vi "FileSync.Read Config.vi"(8 "error in (no error)":errorcluster, 9 "Dialog":bool, 10 "Config File":path, 11 "File.Sync in":refnum<class "File.Sync.lvclass">) -> (0 "error out":errorcluster, 1 "SyncItems":T1[](array[typedef]), 2 "Saved":bool, 3 "File.Sync out":refnum<class "File.Sync.lvclass">)   [LabVIEW 2024, in "KATE_Lib.lvlib" / "File Utils.lvlib" / "File.Sync.lvclass"]
uses:
  File.Sync.lvclass
  File.Sync Item Record.ctl
  File.Sync.lvclass/File.Sync.ctl
  File Utils.lvlib
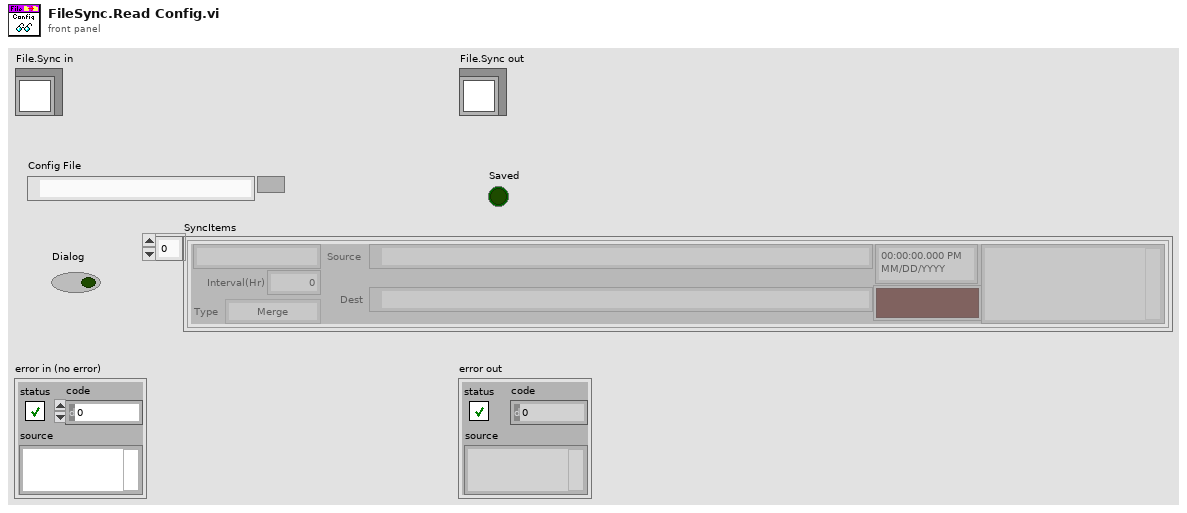
[diagram p1: front panel]
types:
  T1 = typedef "KATE_Lib.lvlib/File Utils.lvlib/File.Sync.lvclass/File.Sync Item Record.ctl" = cluster{"Name":string, "Interval":dbl, "Source":path, "Dest":path, "LastSync":timestamp, "Status":string, "Error":bool, "Type":enum16{"Merge", "Match"}}
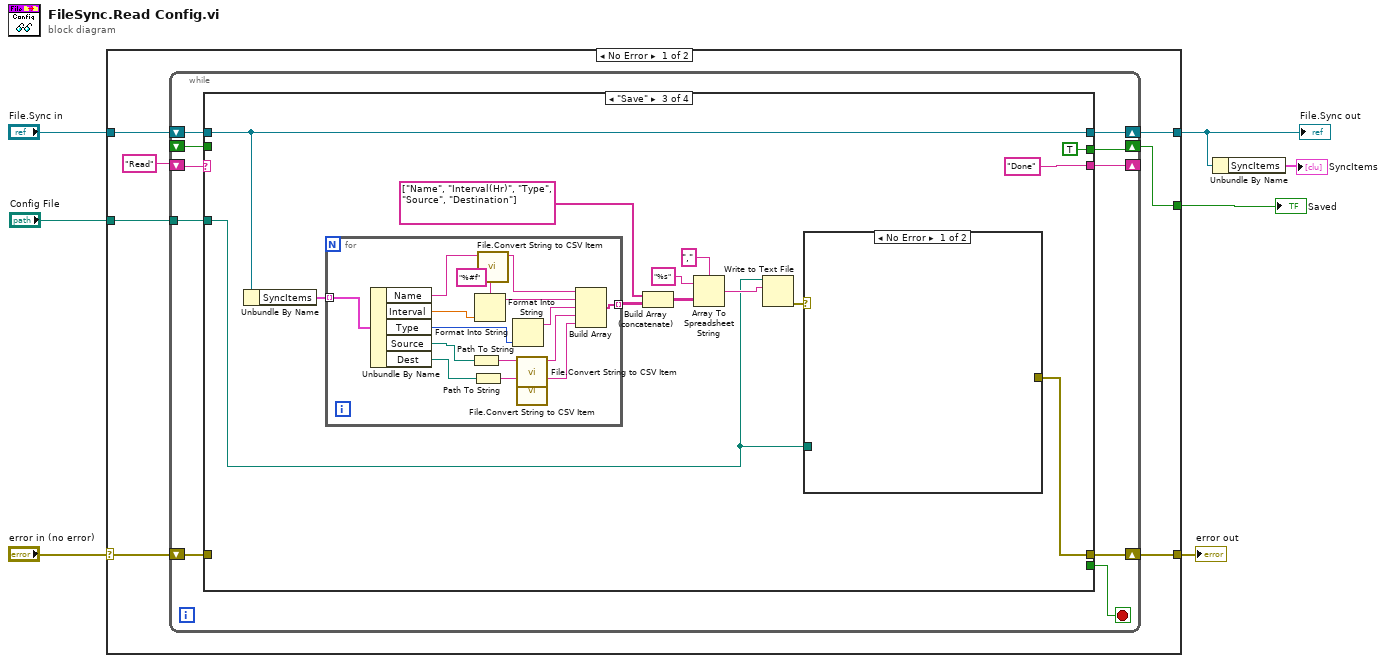
[diagram p0: block diagram]
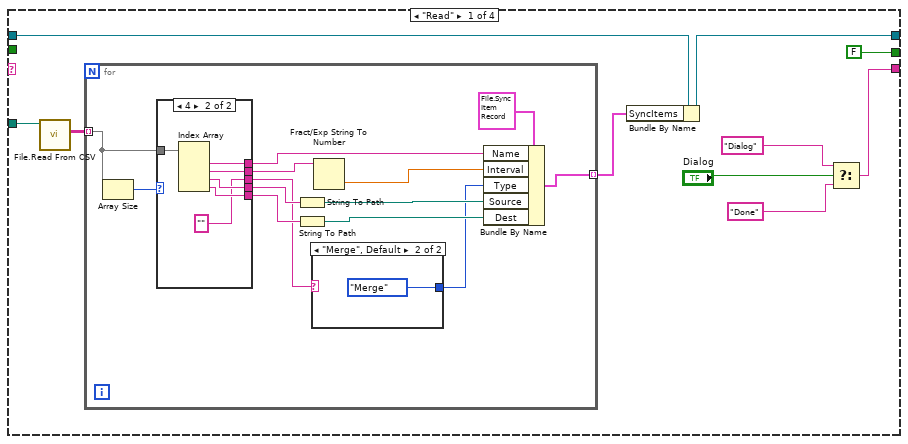
[diagram p2: hidden frame]
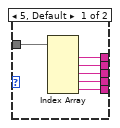
[diagram p3: hidden frame]
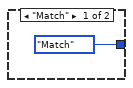
[diagram p4: hidden frame]
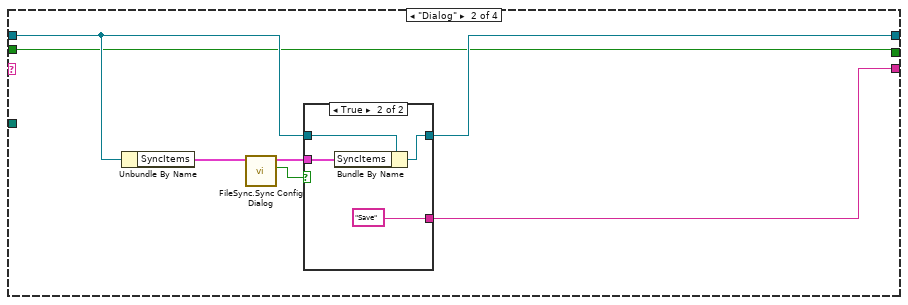
[diagram p5: hidden frame]
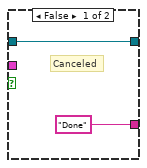
[diagram p6: hidden frame]
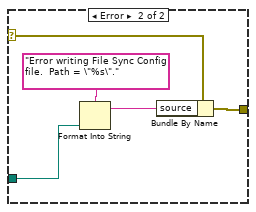
[diagram p7: hidden frame]
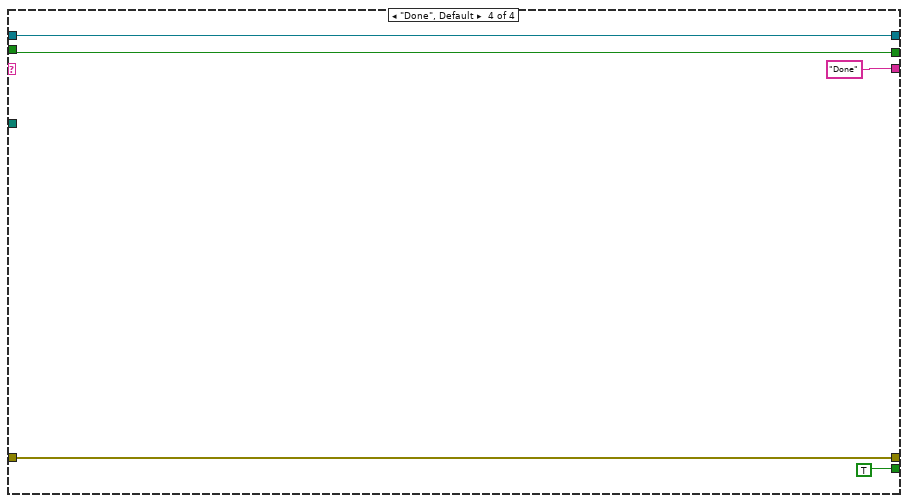
[diagram p8: hidden frame]
diagram:
  n1 = case shown="No Error" "error in (no error)" {
    selector: "error in (no error)" -> [w10 w114]
    tunnel: [w9 w114] -> w6
    tunnel: [w12 w113] -> w2
    tunnel: "File.Sync in" -> [w13 w113]
    tunnel: "Config File" -> [w14 _]
    tunnel: [w8 _] -> w3
    frame No Error {
      n2 = while {
        tunnel: w14 -> [w24]
        shift-right: [w22] -> w12
        shift-left: w13 -> [w23]
        shift-right: [w19] -> _
        shift-left: "Read" -> [w20]
        shift-right: [w18] -> w9
        shift-left: w10 -> [w21]
        shift-right: [w15] -> w8
        shift-left: _ -> [w16]
        stop <- w17 stop-if-true
        n3 = case shown="\"Save\"" w20 {
          tunnel: w24 -> [w34 _ w77 _]
          tunnel: w23 -> [w32 w65 w87 w112]
          tunnel: [w31 w64 w87 w112] -> w22
          tunnel: w21 -> [_ _ _ w110]
          tunnel: [w26 w63 "Done" "Done"] -> w19
          tunnel: [_ _ w76 w110] -> w18
          tunnel: [_ _ _ TRUE] -> w17
          tunnel: w16 -> [_ w62 _ w108]
          tunnel: [FALSE w62 TRUE w108] -> w15
          frame "Read" {
            n4 = call "File.Read From CSV.vi"("File"=w34) -> ("Data"=w33:string[][])  [unwired: 8 in, 2 out]
            n5 = for {
              tunnel: w33 -> [w36] mode=indexing
              tunnel: [w42] -> w30 mode=indexing
              n6 = Array Size(array=w36) -> (size(s)=w35:i32)
              n7 = case shown="4" w35 {
                tunnel: [w53 w59] -> w46
                tunnel: [w52 w58] -> w45
                tunnel: [w51 w55] -> w41
                tunnel: [w50 w56] -> w40
                tunnel: [w49 ""] -> w39
                tunnel: w36 -> [w48 w57]
                frame 5, Default {
                  n8 = Index Array(array=w48) -> (element #1=w53:string, element #2=w52:string, element #3=w49:string, element #4=w50:string, element #5=w51:string)  [unwired: 5 in]
                }
                frame 4 {
                  n9 = Index Array(array=w57) -> (element #1=w59:string, element #2=w58:string, element #3=w56:string, element #4=w55:string)  [unwired: 4 in]
                }
              }
              n10 = String To Path(string=w40) -> (path=w44:path)
              n11 = String To Path(string=w41) -> (path=w43:path)
              n12 = case shown="\"Merge\", Default" w39 {
                tunnel: [enum16{"Merge", "Match"}."Match" ("Type") enum16{"Merge", "Match"}."Merge" ("Type")] -> w38
                frame "Match" {
                }
                frame "Merge", Default {
                }
              }
              n13 = Fract/Exp String To Number(string=w45) -> (number=w37:dbl)  [unwired: 3 in, 1 out]
              n14 = Bundle By Name(cluster=T1 {"Name"="", "Interval"=0.0, "Source"=path "", "Dest"=path "", "LastSync"=timestamp(0 s since 1904-01-01), "Status"="", "Error"=FALSE, "Type"=enum."Merge"} ("SyncItem"), "Name"=w46, "Interval"=w37, "Type"=w38, "Source"=w44, "Dest"=w43) -> (w42:T1)
            }
            n15 = Bundle By Name(cluster=w32, "SyncItems"=w30) -> (w31:refnum<class "File.Sync.lvclass">)
            n16 = Select(t="Dialog", s="Dialog", f="Done") -> (s? t:f=w26:string)
          }
          frame "Dialog" {
            n17 = Unbundle By Name(w65) -> ("SyncItems"=w68:T1[])
            n18 = call "FileSync.Sync Config Dialog.vi"("Sync Config"=w68) -> ("OK"=w67:bool, "Sync Config Out"=w66:T1[])  [unwired: 9 in]
            n19 = case shown="True" w67 {
              tunnel: w66 -> [_ w73]
              tunnel: w65 -> [w70 w74]
              tunnel: [w70 w72] -> w64
              tunnel: ["Done" "Save"] -> w63
              frame False {
                # "Canceled"
              }
              frame True {
                n20 = Bundle By Name(cluster=w74, "SyncItems"=w73) -> (w72:refnum<class "File.Sync.lvclass">)
              }
            }
          }
          frame "Save" {
            n21 = Unbundle By Name(w87) -> ("SyncItems"=w85:T1[])
            n22 = for {
              tunnel: w85 -> [w107] mode=indexing
              tunnel: [w105] -> w83 mode=indexing
              n23 = Unbundle By Name(w107) -> ("Name"=w103:string, "Interval"=w98:dbl, "Type"=w94:enum16{"Merge", "Match"}, "Source"=w95:path, "Dest"=w106:path)
              n24 = Path To String(path=w95) -> (string=w99:string)
              n25 = Path To String(path=w106) -> (string=w104:string)
              n26 = Format Into String(format string="%#f", w98) -> (resulting string=w97:string)  [unwired: 2 in, 1 out]
              n27 = call "File.Convert String to CSV Item.vi"("String"=w103) -> ("String Out"=w102:string)  [unwired: 10 in]
              n28 = Format Into String(w94) -> (resulting string=w93:string)  [unwired: 3 in, 1 out]
              n29 = call "File.Convert String to CSV Item.vi"("String"=w99) -> ("String Out"=w101:string)  [unwired: 10 in]
              n30 = call "File.Convert String to CSV Item.vi"("String"=w104) -> ("String Out"=w100:string)  [unwired: 10 in]
              n31 = Build Array(w102, w97, w93, w101, w100) -> (w105:string[])
            }
            n32 = Build Array (concatenate)(string[] ["Name", "Interval(Hr)", "Type", "Source", "Destination"], w83) -> (w82:string[][])
            n33 = Array To Spreadsheet String(delimiter (Tab)=",", array=w82, 3:"%s" ("format string")) -> (spreadsheet string=w79:string)
            n34 = Write to Text File(file (use dialog)=w77, text=w79) -> (error out=w78:errorcluster)  [unwired: 2 in, 2 out]
            n35 = case shown="No Error" w78 {
              selector: w78 -> [_ w92]
              tunnel: w77 -> [_ w89]
              tunnel: [_ w91] -> w76
              frame No Error {
              }
              frame Error {
                n36 = Format Into String(format string="Error writing File Sync Config file.  Path = \"%s\".", w89) -> (resulting string=w88:string)  [unwired: 2 in, 1 out]
                n37 = Bundle By Name(cluster=w92, "source"=w88) -> (w91:errorcluster)
              }
            }
          }
          frame "Done", Default {
          }
        }
      }
    }
    frame Error {
    }
  }
  "error out" <- w6
  "File.Sync out" <- w2
  "Saved" <- w3
  n38 = Unbundle By Name(w2) -> ("SyncItems"=→"SyncItems":T1[])
